vi "选项卡控件.vi"() -> ()   [LabVIEW 2018]
panel:
  in  "索引":i32
  in  "确定按钮":bool
  out "选项卡控件":enum32{"a 1", "b"}(tab)
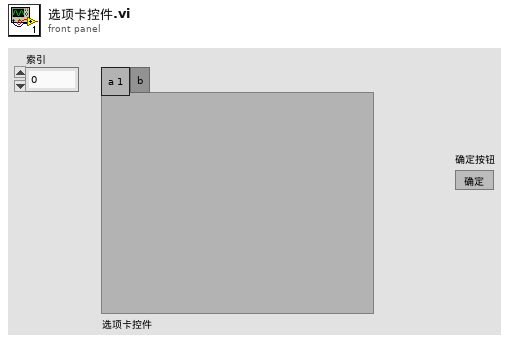
[diagram p1: front panel]
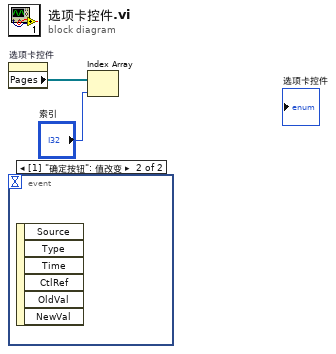
[diagram p0: block diagram]
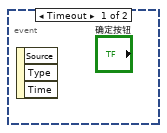
[diagram p2: hidden frame]
diagram:
  n1 = property on="选项卡控件" class="TabCtl (严格)"() -> ("Pages"=w2:refnum<vi>[])  [unwired: 2 in, 2 out]
  n2 = event shown="[1] \"确定按钮\": 值改变" {
    selector: _ -> [_ _]
    dyn-events: _ -> [_ _]
    timeout: _ -> [_ _]
    event Timeout {
      n3 = event-data() -> ()  [unwired: 1 in, 3 out]
    }
    event "确定按钮": Value Change {
      n4 = event-data() -> ()  [unwired: 1 in, 6 out]
    }
  }
  n5 = Index Array(array=w2, index="索引") -> ()  [unwired: 1 out]
